vi "return phase.vi"(11 "VISA resource name":refnum<visa-resource-name>) -> (3 "return phase":string)   [LabVIEW 2014]
panel:
  out "VISA resource name out":refnum<visa-resource-name>
  out "error out":errorcluster
  in  "error in (no error)":errorcluster
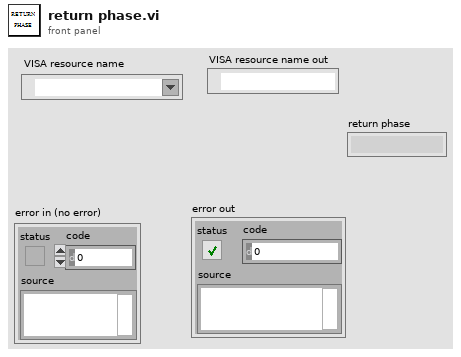
[diagram p1: front panel]
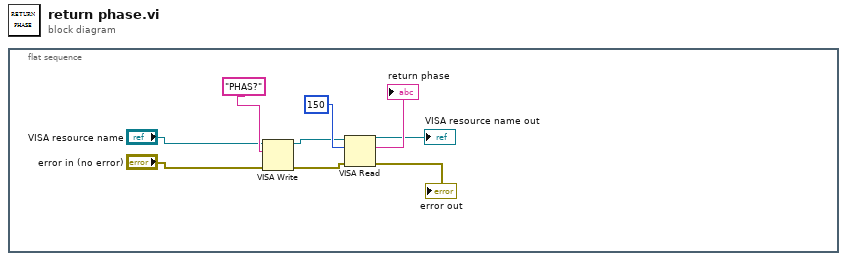
[diagram p0: block diagram]
diagram:
  n1 = flat-sequence {
    frame #0 {
      n2 = VISA Write(VISA resource name="VISA resource name", write buffer="PHAS?" ("format string"), error in (no error)="error in (no error)") -> (VISA resource name out=w4:refnum<visa-resource-name>, error out=w3:errorcluster)  [unwired: 1 out]
      n3 = VISA Read(VISA resource name=w4, byte count=u32 150, error in (no error)=w3) -> (VISA resource name out=→"VISA resource name out":refnum<visa-resource-name>, read buffer=→"return phase":string, error out=→"error out":errorcluster)  [unwired: 1 out]
    }
  }
